vi "Get Tree Activate Node Name.vi"(8 "error in (no error)":errorcluster, 11 "MyTreeAPI in":refnum<class "MyTreeAPI.lvclass">) -> (0 "error out":errorcluster, 2 "Cell String":string, 3 "MyTreeAPI out":refnum<class "MyTreeAPI.lvclass">)   [LabVIEW 2015, in "MyTreeAPI.lvclass"]
uses:
  MyTreeAPI.lvclass
  MyTreeAPI.lvclass/MyTreeAPI.ctl
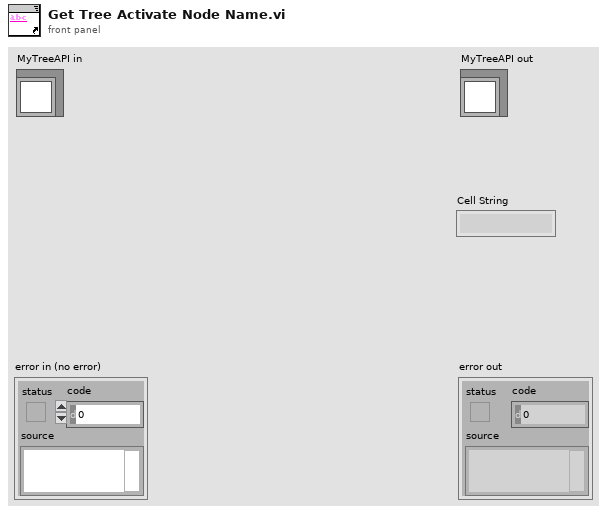
[diagram p1: front panel]
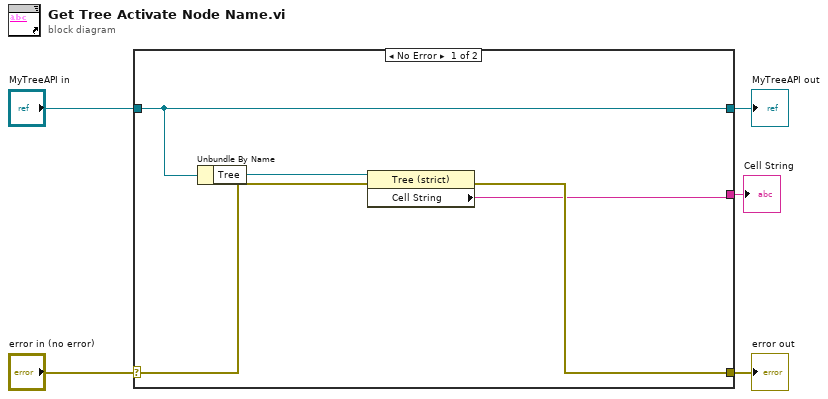
[diagram p0: block diagram]
diagram:
  n1 = case shown="No Error" "error in (no error)" {
    selector: "error in (no error)" -> [w8 w12]
    tunnel: [w7 w12] -> w4
    tunnel: [w10 w11] -> w2
    tunnel: "MyTreeAPI in" -> [w10 w11]
    tunnel: [w6 _] -> w1
    frame No Error {
      n2 = Unbundle By Name(w10) -> ("Tree"=w9:refnum<vi>)
      n3 = property class="Tree (strict)"(reference=w9, error in=w8) -> (error out=w7:errorcluster, "Cell String"=w6:string)  [unwired: 1 out]
    }
    frame Error {
    }
  }
  "error out" <- w4
  "MyTreeAPI out" <- w2
  "Cell String" <- w1
